vi "ROI_plot_XY_embryo_positions.vi"(4 "Pos 2 saved":bool, 5 "REF positions":dbl[][](array[numeric]), 6 "Pos 1 saved":bool, 7 "XYGraph Refnum":refnum<vi>, 8 "Embryo position 2":cluster{"x(um)":dbl, "y(um)":dbl, "z(um)":dbl}, 9 "Embryo position 1":cluster{"x(um)":dbl, "y(um)":dbl, "z(um)":dbl}, 10 "error in":errorcluster, 11 "XY positions":dbl[][](array[numeric])) -> (0 "XY graph":cluster{dbl[], dbl[]}[](array[cluster]), 3 "error out":errorcluster)   [LabVIEW 2015]
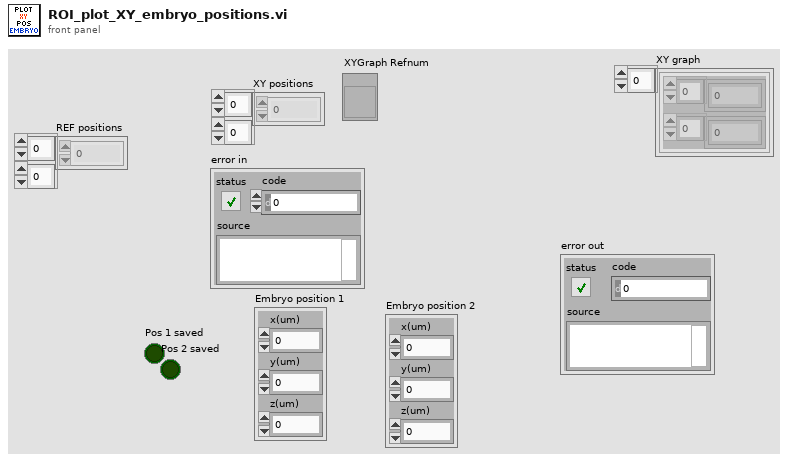
[diagram p1: front panel]
types:
  T1 = typedef "LVRangeTypeDef.ctl" = cluster{"Minimum":dbl, "Maximum":dbl, "Increment":dbl, "Minor Increment":dbl, "Start":dbl}
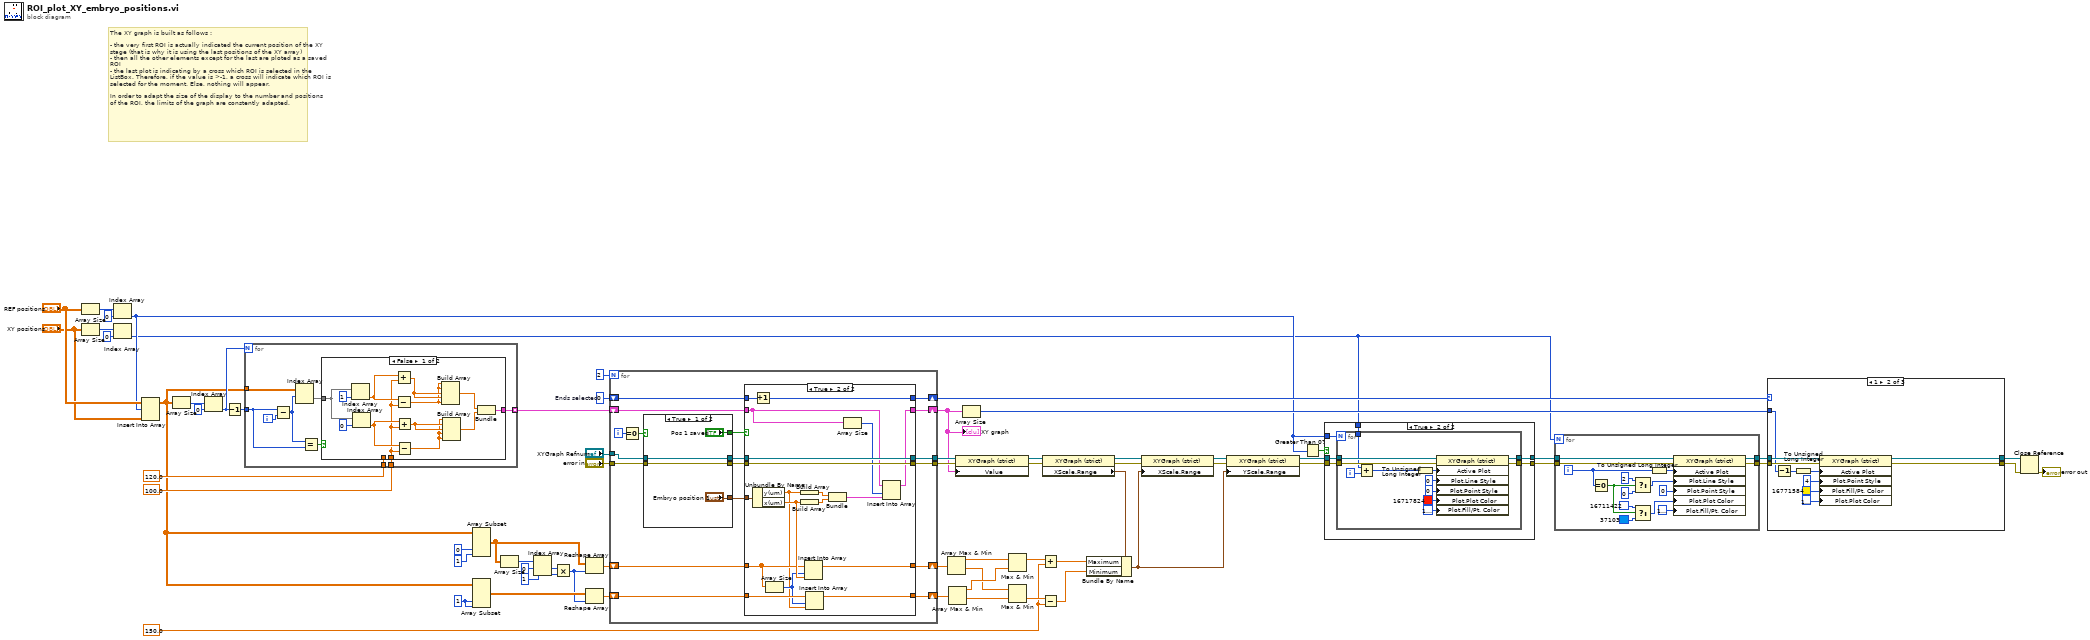
[diagram p0: block diagram]
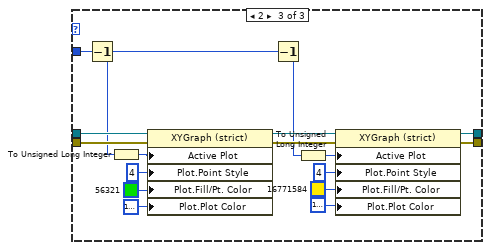
[diagram p4: hidden frame]
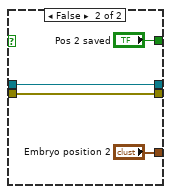
[diagram p5: hidden frame]
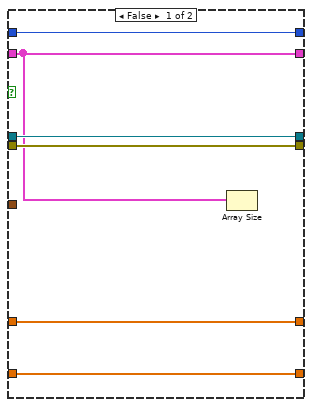
[diagram p6: hidden frame]
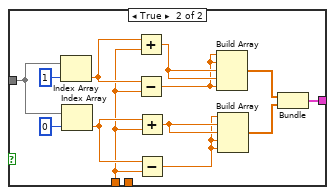
[diagram p7: hidden frame]
diagram:
  w42 = 150.0 ("y")
  w41 = 0  # Ends selected
  w60 = 1 ("index")
  # "The XY graph is built as follows :\n\n- the very first ROI is actually indicated the current position of the XY stage (that is why it is using the last positions of the XY array)\n- then all the other elements except for the last are ploted as a saved ROI\n- the last plot is indicating by a cross which ROI is selected in the ListBox. Therefore, if the value is >-1, a cross will indicate which ROI is selected for the moment. Else, nothing will appear.\n\nIn order to adapt the size of the display to the number and positions of the ROI, the limits of the graph are constently adapted."
  n1 = Array Size(array="XY positions") -> (size(s)=w15:i32[])
  n2 = Array Size(array="REF positions") -> (size(s)=w16:i32[])
  n3 = Index Array(array=w15, index=0) -> (element=w1:i32)
  n4 = Index Array(array=w16, index=0) -> (element=w2:i32)
  n5 = Insert Into Array(array="REF positions", index (row)=w2, new element="XY positions") -> (w43:dbl[][])  [unwired: 1 in]
  n6 = Array Size(array=w43) -> (size(s)=w67:i32[])
  n7 = Index Array(array=w67, index=0) -> (element=w50:i32)
  n8 = Decrement(x=w50) -> (x-1=w49:i32)
  n9 = for {
    N: w50 -> [_]
    tunnel: w43 -> [w76]
    tunnel: [w74] -> w21 mode=indexing
    tunnel: w49 -> [w70]
    tunnel: 120.0 ("y") -> [w69]
    tunnel: 100.0 ("y") -> [w68]
    i -> [w72]
    n10 = Subtract(x=w70, y=w72) -> (x-y=w71:i32)
    n11 = Index Array(array=w76, index (row)=w71) -> (element=w75:dbl[])  [unwired: 1 in]
    n12 = Equal?(x=w71, y=w70) -> (x = y?=w73:bool)
    n13 = case shown="False" w73 {
      tunnel: w75 -> [w79 w91]
      tunnel: [w78 w92] -> w74
      tunnel: w69 -> [_ w90]
      tunnel: w68 -> [w77 _]
      frame False {
        n14 = Index Array(array=w79, index=1 ("index (row)")) -> (element=w87:dbl)
        n15 = Index Array(array=w79, index=0 ("index (row)")) -> (element=w84:dbl)
        n16 = Add(x=w87, y=w77) -> (x+y=w86:dbl)
        n17 = Subtract(x=w87, y=w77) -> (x-y=w85:dbl)
        n18 = Add(x=w84, y=w77) -> (x+y=w83:dbl)
        n19 = Subtract(x=w84, y=w77) -> (x-y=w82:dbl)
        n20 = Build Array(w85, w85, w86, w86, w85) -> (w81:dbl[])
        n21 = Build Array(w82, w83, w83, w82, w82) -> (w80:dbl[])
        n22 = Bundle(w81, w80) -> (w78:cluster{dbl[], dbl[]})  [unwired: 1 in]
      }
      frame True {
        n23 = Index Array(array=w91, index=1 ("index (row)")) -> (element=w100:dbl)
        n24 = Index Array(array=w91, index=0 ("index (row)")) -> (element=w97:dbl)
        n25 = Add(x=w100, y=w90) -> (x+y=w99:dbl)
        n26 = Subtract(x=w100, y=w90) -> (x-y=w98:dbl)
        n27 = Add(x=w97, y=w90) -> (x+y=w96:dbl)
        n28 = Subtract(x=w97, y=w90) -> (x-y=w95:dbl)
        n29 = Build Array(w98, w98, w99, w99, w98) -> (w94:dbl[])
        n30 = Build Array(w95, w96, w96, w95, w95) -> (w93:dbl[])
        n31 = Bundle(w94, w93) -> (w92:cluster{dbl[], dbl[]})  [unwired: 1 in]
      }
    }
  }
  n32 = Array Subset(array=w43, index (col)=0 ("index"), length (col)=1 ("length")) -> (w34:dbl[][])  [unwired: 2 in]
  n33 = Array Subset(array=w43, index (col)=w60, length (col)=w60) -> (w28:dbl[][])  [unwired: 2 in]
  n34 = Array Size(array=w34) -> (size(s)=w33:i32[])
  n35 = Index Array(array=w33, index #1=0 ("index"), index #2=1 ("index")) -> (element #1=w30:i32, element #2=w29:i32)
  n36 = Multiply(x=w30, y=w29) -> (x*y=w27:i32)
  n37 = Reshape Array(w34, w27) -> (w35:dbl[])
  n38 = Reshape Array(w28, w27) -> (w26:dbl[])
  n39 = for {
    N: 2 -> [_]
    tunnel: "error in" -> [w118]
    tunnel: "XYGraph Refnum" -> [w113]
    tunnel: [w112] -> w36
    tunnel: [w111] -> w37
    shift-right: [w109] -> w12
    shift-left: w41 -> [w110]
    shift-right: [w107] -> w18
    shift-left: w21 -> [w108]
    shift-right: [w104] -> w25
    shift-left: w35 -> [w105]
    shift-right: [w103] -> w24
    shift-left: w26 -> [w106]
    i -> [w116]
    n40 = Equal To 0?(x=w116) -> (x = 0?=w115:bool)
    n41 = case shown="True" w115 {
      tunnel: ["Pos 1 saved" "Pos 2 saved"] -> w120
      tunnel: ["Embryo position 1" "Embryo position 2"] -> w119
      tunnel: w118 -> [w122 w126]
      tunnel: [w122 w126] -> w117
      tunnel: [w121 w125] -> w114
      tunnel: w113 -> [w121 w125]
      frame True {
      }
      frame False {
      }
    }
    n42 = case shown="True" w120 {
      tunnel: w117 -> [w132 w146]
      tunnel: w119 -> [_ w150]
      tunnel: w114 -> [w133 w147]
      tunnel: [w132 w146] -> w112
      tunnel: [w133 w147] -> w111
      tunnel: w110 -> [w134 w149]
      tunnel: [w134 w148] -> w109
      tunnel: w108 -> [w131 w136]
      tunnel: [w131 w138] -> w107
      tunnel: w105 -> [w130 w143]
      tunnel: w106 -> [w129 w142]
      tunnel: [w130 w144] -> w104
      tunnel: [w129 w139] -> w103
      frame False {
        n43 = Array Size(array=w131) -> ()  [unwired: 1 out]
      }
      frame True {
        n44 = Unbundle By Name(w150) -> ("y(um)"=w140:dbl, "x(um)"=w145:dbl)
        n45 = Increment(x=w149) -> (x+1=w148:i32)
        n46 = Array Size(array=w143) -> (size(s)=w141:i32)
        n47 = Build Array(w140) -> (w152:dbl[])
        n48 = Build Array(w145) -> (w151:dbl[])
        n49 = Insert Into Array(array=w143, index=w141, new element=w145) -> (w144:dbl[])
        n50 = Insert Into Array(array=w142, index=w141, new element=w140) -> (w139:dbl[])
        n51 = Bundle(w152, w151) -> (w135:cluster{dbl[], dbl[]})  [unwired: 1 in]
        n52 = Array Size(array=w136) -> (size(s)=w137:i32)
        n53 = Insert Into Array(array=w136, index=w137, new element=w135) -> (w138:cluster{dbl[], dbl[]}[])
      }
    }
  }
  "XY graph" <- w18
  n54 = Array Max & Min(array=w25) -> (max value=w59:dbl, min value=w56:dbl)  [unwired: 2 out]
  n55 = Array Max & Min(array=w24) -> (max value=w58:dbl, min value=w57:dbl)  [unwired: 2 out]
  n56 = property class="XYGraph (strict)"(reference=w37, error in=w36, "Value"=w18) -> (reference out=w23:refnum<vi>, error out=w22:errorcluster)
  n57 = Array Size(array=w18) -> (size(s)=w13:i32)
  n58 = Max & Min(x=w59, y=w58) -> (max(x,y)=w55:dbl)  [unwired: 1 out]
  n59 = Max & Min(x=w56, y=w57) -> (min(x,y)=w53:dbl)  [unwired: 1 out]
  n60 = Add(x=w55, y=w42) -> (x+y=w54:dbl)
  n61 = Subtract(x=w53, y=w42) -> (x-y=w52:dbl)
  n62 = property class="XYGraph (strict)"(reference=w23, error in=w22) -> (reference out=w48:refnum<vi>, error out=w47:errorcluster, "XScale.Range"=w63:T1)
  n63 = Bundle By Name(cluster=w63, "Maximum"=w54, "Minimum"=w52) -> (w51:T1)
  n64 = property class="XYGraph (strict)"(reference=w48, error in=w47, "XScale.Range"=w51) -> (reference out=w65:refnum<vi>, error out=w64:errorcluster)
  n65 = property class="XYGraph (strict)"(reference=w65, error in=w64, "YScale.Range"=w51) -> (reference out=w6:refnum<vi>, error out=w5:errorcluster)
  n66 = Greater Than 0?(x=w2) -> (x > 0?=w11:bool)
  n67 = case shown="True" w11 {
    tunnel: w6 -> [w154 w160]
    tunnel: w5 -> [w153 w159]
    tunnel: [w154 w158] -> w4
    tunnel: [w153 w157] -> w3
    tunnel: w2 -> [_ w156]
    tunnel: w1 -> [_ w155]
    frame False {
    }
    frame True {
      n68 = for {
        N: w156 -> [_]
        tunnel: w160 -> [w166]
        tunnel: w159 -> [w167]
        tunnel: [w172] -> w158
        tunnel: [w171] -> w157
        tunnel: w155 -> [w161]
        i -> [w163]
        n69 = Add(x=w161, y=w163) -> (x+y=w162:i32)
        n70 = To Unsigned Long Integer(number=w162) -> (unsigned 32bit integer=w170:u32)
        n71 = property class="XYGraph (strict)"(reference=w166, error in=w167, "Active Plot"=w170, "Plot.Line Style"=u8 0 ("Plot.Plot Color"), "Plot.Point Style"=u8 0, "Plot.Plot Color"=u32 16717824, "Plot.Fill/Pt. Color"=u32 16777216) -> (reference out=w172:refnum<vi>, error out=w171:errorcluster)
      }
    }
  }
  n72 = for {
    N: w1 -> [_]
    tunnel: w4 -> [w187]
    tunnel: w3 -> [w186]
    tunnel: [w184] -> w8
    tunnel: [w183] -> w7
    i -> [w173]
    n73 = Equal To 0?(x=w173) -> (x = 0?=w179:bool)
    n74 = Select(t=u8 2, s=w179, f=u8 0 ("Plot.Plot Color")) -> (s? t:f=w180:u8)
    n75 = Select(t=u32 16711422, s=w179, f=u32 37103) -> (s? t:f=w176:u32)
    n76 = To Unsigned Long Integer(number=w173) -> (unsigned 32bit integer=w185:u32)
    n77 = property class="XYGraph (strict)"(reference=w187, error in=w186, "Active Plot"=w185, "Plot.Line Style"=w180, "Plot.Point Style"=u8 0, "Plot.Plot Color"=w176, "Plot.Fill/Pt. Color"=u32 16777216) -> (reference out=w184:refnum<vi>, error out=w183:errorcluster)
  }
  n78 = case shown="1" w12 {
    tunnel: w8 -> [w189 w198 w214]
    tunnel: w7 -> [w188 w197 w212]
    tunnel: w13 -> [_ w196 w216]
    tunnel: [w189 w194 w211] -> w20
    tunnel: [w188 w193 w204] -> w19
    frame 0, Default {
    }
    frame 1 {
      n79 = Decrement(x=w196) -> (x-1=w195:i32)
      n80 = To Unsigned Long Integer(number=w195) -> (unsigned 32bit integer=w191:u32)
      n81 = property class="XYGraph (strict)"(reference=w198, error in=w197, "Active Plot"=w191, "Plot.Point Style"=u8 4, "Plot.Fill/Pt. Color"=u32 16771584, "Plot.Plot Color"=u32 16777216) -> (reference out=w194:refnum<vi>, error out=w193:errorcluster)
    }
    frame 2 {
      n82 = Decrement(x=w216) -> (x-1=w207:i32)
      n83 = To Unsigned Long Integer(number=w207) -> (unsigned 32bit integer=w213:u32)
      n84 = property class="XYGraph (strict)"(reference=w214, error in=w212, "Active Plot"=w213, "Plot.Point Style"=u8 4, "Plot.Fill/Pt. Color"=u32 56321, "Plot.Plot Color"=u32 16777216) -> (reference out=w210:refnum<vi>, error out=w209:errorcluster)
      n85 = Decrement(x=w207) -> (x-1=w206:i32)
      n86 = To Unsigned Long Integer(number=w206) -> (unsigned 32bit integer=w205:u32)
      n87 = property class="XYGraph (strict)"(reference=w210, error in=w209, "Active Plot"=w205, "Plot.Point Style"=u8 4, "Plot.Fill/Pt. Color"=u32 16771584, "Plot.Plot Color"=u32 16777216) -> (reference out=w211:refnum<vi>, error out=w204:errorcluster)
    }
  }
  n88 = Close Reference(reference=w20, error in (no error)=w19) -> (error out=→"error out":errorcluster)
